vi "计算合并值.vi"(2 "数值H":u8, 3 "数值L":u8) -> (16 "合并数值":i16)   [LabVIEW 2016]
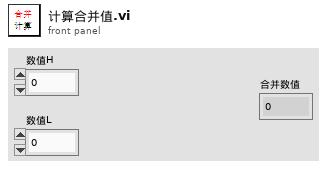
[diagram p1: front panel]
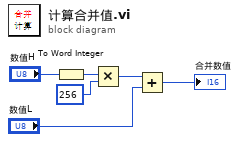
[diagram p0: block diagram]
diagram:
  n1 = To Word Integer(number="数值H") -> (16bit integer=w3:i16)
  n2 = Multiply(x=w3, y=256) -> (x*y=w1:i32)
  n3 = Add(x=w1, y="数值L") -> (x+y=→"合并数值":i32)
